vi "Dynamic Call Main VI.vi"   [LabVIEW 2010]
types:
  T1 = typedef "Path InitDynamicVIsPaths__FS.ctl" = cluster{"F4 Operation":path, "F4 Alarms":path, "F4 Inputs":path, "F4 Outputs":path, "F4 PID Sets":path, "F4 Cascade":path, "F4 Current Step":path, "Profile SubPanel":path, "Profile Editor":path, "MainVI":path, "Profile Control":path, "Synergy Control":path, "Driver Server":path}
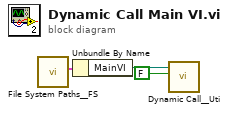
[diagram p0: block diagram]
diagram:
  n1 = call "File System Paths__FS.vi"() -> ("DynamicVIs"=w3:T1)  [unwired: 9 in, 2 out]
  n2 = Unbundle By Name(w3) -> ("MainVI"=w2:path)
  n3 = call "Dynamic Call__Uti.vi"("open front panel? (T)"=FALSE, "vi path"=w2) -> ()  [unwired: 9 in, 1 out]
